vi "DisplacementSetSensorRawValue.vi"(9 "Value":i32, 10 "Sensor":u8, 11 "DisplacementSample in":T1) -> (3 "DisplacementSample out":T1)   [LabVIEW 2016]
uses:
  DisplacementSample.ctl
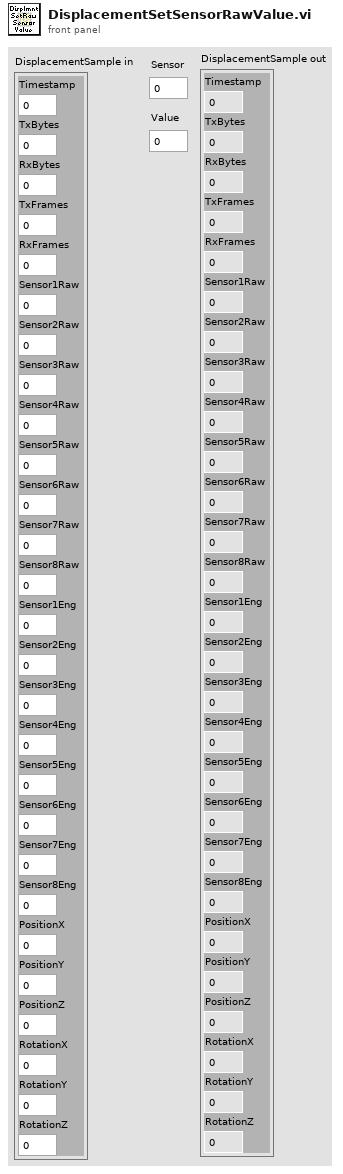
[diagram p1: front panel]
types:
  T1 = typedef "DisplacementSample.ctl" = cluster{"Timestamp":u64, "TxBytes":u64, "RxBytes":u64, "TxFrames":u64, "RxFrames":u64, "Sensor1Raw":i32, "Sensor2Raw":i32, "Sensor3Raw":i32, "Sensor4Raw":i32, "Sensor5Raw":i32, "Sensor6Raw":i32, "Sensor7Raw":i32, "Sensor8Raw":i32, "Sensor1Eng":sgl, "Sensor2Eng":sgl, "Sensor3Eng":sgl, "Sensor4Eng":sgl, "Sensor5Eng":sgl, "Sensor6Eng":sgl, "Sensor7Eng":sgl, "Sensor8Eng":sgl, "PositionX":sgl, "PositionY":sgl, "PositionZ":sgl, "RotationX":sgl, "RotationY":sgl, "RotationZ":sgl}
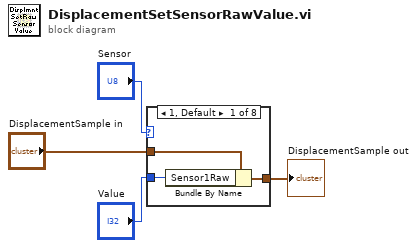
[diagram p0: block diagram]
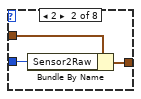
[diagram p2: hidden frame]
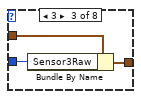
[diagram p3: hidden frame]
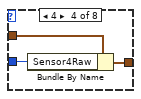
[diagram p4: hidden frame]
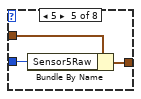
[diagram p5: hidden frame]
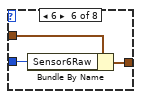
[diagram p6: hidden frame]
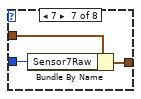
[diagram p7: hidden frame]
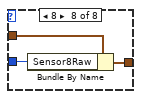
[diagram p8: hidden frame]
diagram:
  n1 = case shown="1, Default" "Sensor" {
    tunnel: "DisplacementSample in" -> [w7 w10 w13 w16 w19 w22 w25 w28]
    tunnel: [w6 w9 w12 w15 w18 w21 w24 w27] -> w2
    tunnel: "Value" -> [w5 w8 w11 w14 w17 w20 w23 w26]
    frame 1, Default {
      n2 = Bundle By Name(cluster=w7, "Sensor1Raw"=w5) -> (w6:T1)
    }
    frame 2 {
      n3 = Bundle By Name(cluster=w10, "Sensor2Raw"=w8) -> (w9:T1)
    }
    frame 3 {
      n4 = Bundle By Name(cluster=w13, "Sensor3Raw"=w11) -> (w12:T1)
    }
    frame 4 {
      n5 = Bundle By Name(cluster=w16, "Sensor4Raw"=w14) -> (w15:T1)
    }
    frame 5 {
      n6 = Bundle By Name(cluster=w19, "Sensor5Raw"=w17) -> (w18:T1)
    }
    frame 6 {
      n7 = Bundle By Name(cluster=w22, "Sensor6Raw"=w20) -> (w21:T1)
    }
    frame 7 {
      n8 = Bundle By Name(cluster=w25, "Sensor7Raw"=w23) -> (w24:T1)
    }
    frame 8 {
      n9 = Bundle By Name(cluster=w28, "Sensor8Raw"=w26) -> (w27:T1)
    }
  }
  "DisplacementSample out" <- w2
